vi "dvotAFTConstants.vi"() -> ()   [LabVIEW 2012]
panel:
  out "CELL_PARAM_A":i32=5
  out "RMR0":i32=4
  out "CL_WT_PCT":i32=3
  out "OH_PFU":i32=2
  out "CL_PFU":i32=1
  out "ETCH_PIT_LENGTH":i32
  out "KPAR_NOT_USED":i32=-1
  out "ETCH_50M_20C_20S":i32=1
  out "ETCH_55M_21C_20S":i32
  out "KETCHAM_2003":i32=3
  out "DONELICK_ET_AL_1999":i32=2
  out "KETCHAM_ET_AL_2007_55":i32=1
  out "KETCHAM_ET_AL_2007_50":i32
  out "PROJ_NOT_USED":i32=-1
  out "CROWLEY_ET_AL_FAP_1991":dbl=3.0
  out "LASLETT_ET_AL_DUR_1987":dbl=2.0
  out "KETCHAM_ET_AL_1999":i32=1
  out "KETCHAM_ET_AL_2007":i32
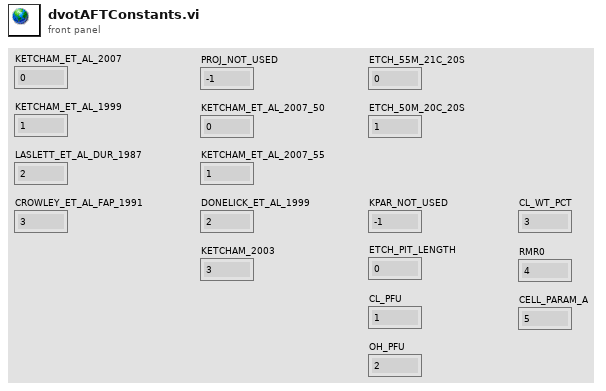
[diagram p1: front panel]
diagram:
